vi "Begin.vi"(8 "error in":errorcluster) -> (0 "error out":errorcluster)   [LabVIEW 2014]
doc: "Called before other user functions, this VI is expected to open initial I/O refnums, load in file data, and do all program initialization. Notice that the <B>error out</B> terminal is simply used for data flow. Wiring it to other structures or subVIs ensures that this VI runs first."
uses:
  <vilib>/Rock Robotics/WPI/DriverStation/WPI_DriverStationRobotMode2.ctl
  <vilib>/Rock Robotics/WPI/Joystick/WPI_JoystickDeviceEnum.ctl
  <vilib>/Rock Robotics/WPI/Solenoid/WPI_SolenoidChannel.ctl
  <vilib>/Rock Robotics/SystemInterfaces/AI/FPGA_AIChannel.ctl
  <vilib>/Rock Robotics/SystemInterfaces/DIO/FPGA_DIOChannel.ctl
  <vilib>/Rock Robotics/WPI/CAN/TalonSRX/WPI_CANTalonSRX_APIControlMode.ctl
  <vilib>/Rock Robotics/WPI/CAN/TalonSRX/WPI_CANTalonSRX_BrakeOverride.ctl
  <vilib>/Rock Robotics/SystemInterfaces/i2clib/i2c_bus.ctl
  <vilib>/Rock Robotics/WPI/AnalogOutput/WPI_AnalogOutputChannel.ctl
  navX-MXP Library/COMMON/TypeDefs/Value TypeDefs/navX Update Rate.ctl
  navX-MXP Library/COMMON/TypeDefs/Value TypeDefs/navX Interface Protocol.ctl
  <vilib>/Rock Robotics/SystemInterfaces/spilib/spi_bus.ctl
  Robot Global Data.vi
  <vilib>/Rock Robotics/WPI/Solenoid/WPI_SolenoidOpenSingle.vi
  <vilib>/Rock Robotics/WPI/Counter/WPI_CounterDigitalInputToDigitalSource.vi
  <vilib>/Rock Robotics/WPI/MotorControl/WPI_MotorControlOpenCANTalonSRX.vi
  <vilib>/Rock Robotics/WPI/Ultrasonic/WPI_SonarSRF04DigitalOpen.vi
  <vilib>/Rock Robotics/WPI/Ultrasonic/WPI_SonarSRF04DigitalRefNum Registry Set.vi
  <vilib>/Rock Robotics/WPI/Compressor/WPI_CompressorGetSetRefNum.vi
  <vilib>/Rock Robotics/WPI/Camera/WPI_CameraWhite Balance Values.ctl
  <vilib>/Rock Robotics/WPI/Camera/WPI_CameraExposure Values.ctl
  <vilib>/Rock Robotics/WPI/Accelerometer/ADXL345 Range.ctl
  <vilib>/Rock Robotics/WPI/Accelerometer/WPI_AccelerometerADXL345 Axes.ctl
  <vilib>/Rock Robotics/WPI/RobotDrive/WPI_RobotDriveOpen2MotorWithExistingMotors.vi
  navX-MXP Library/navX-MXP IMU.lvlib
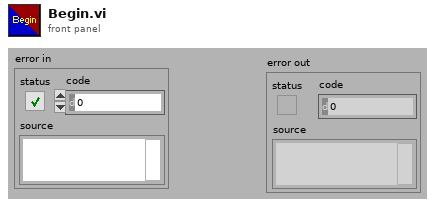
[diagram p1: front panel]
types:
  T1 = typedef "FPGA_DIOChannel.ctl" = enum8{"DIO 0", "DIO 1", "DIO 2", "DIO 3", "DIO 4", "DIO 5", "DIO 6", "DIO 7", "DIO 8", "DIO 9", "DIO MXP 0", "DIO MXP 1", "DIO MXP 2", "DIO MXP 3", "DIO MXP 4", "DIO MXP 5", "DIO MXP 6", "DIO MXP 7", "DIO MXP 8", "DIO MXP 9", "DIO MXP 10", "DIO MXP 11", "DIO MXP 12", "DIO MXP 13", "DIO MXP 14", "DIO MXP 15", "Invalid"}
  T2 = typedef "WPI_AnalogOutputChannel.ctl" = enum8{"AO MXP 0", "AO MXP 1", "Invalid"}
  T3 = typedef "i2c_bus.ctl" = enum16{"I2C On-Board", "I2C MXP", "Invalid"}
  T4 = typedef "FPGA_AIChannel.ctl" = enum8{"AI 0", "AI 1", "AI 2", "AI 3", "AI MXP 0", "AI MXP 1", "AI MXP 2", "AI MXP 3", "Invalid"}
  T5 = typedef "WPI_SolenoidChannel.ctl" = enum8{"Solenoid 0", "Solenoid 1", "Solenoid 2", "Solenoid 3", "Solenoid 4", "Solenoid 5", "Solenoid 6", "Solenoid 7", "Invalid"}
  T6 = typedef "WPI_CANTalonSRX_BrakeOverride.ctl" = enum8{"No Override", "Override to Coast", "Override to Brake"}
  T7 = typedef "WPI_CANTalonSRX_APIControlMode.ctl" = enum8{"Percent VBus", "Speed", "Position", "Slave", "Unchanged / Invalid"}
  T8 = typedef "WPI_JoystickDeviceEnum.ctl" = enum16{"USB 0", "USB 1", "USB 2", "USB 3", "USB 4", "USB 5"}
  T9 = typedef "WPI_DriverStationRobotMode2.ctl" = enum16{"Autonomous Disabled", "Autonomous Enabled", "Teleop Disabled", "Teleop Enabled", "Disconnected", "Finish", "Test Disabled", "Test Enabled", "Emergency Stopped"}
  T10 = typedef "WPI_CameraExposure Values.ctl" = enum16{"Auto", "Flicker-free 50 Hz", "Flicker-free 60 Hz", "Hold current", "Custom"}
  T11 = typedef "WPI_CameraWhite Balance Values.ctl" = enum16{"Auto", "Fixed indoor", "Fixed outdoor 1", "Fixed outdoor 2", "Fixed fluorescent 1", "Fixed fluorescent 2", "Hold current", "Custom"}
  T12 = typedef "WPI_CameraDevRef.ctl" = cluster{"Camera Address":string, "CameraStatus":errorcluster}
  T13 = typedef "WPI_SolenoidDevRef.ctl" = cluster{"DevStatus":errorcluster, "Pneumatics Control Module":u8, "Forward Solenoid Channel":T5, "Reverse Solenoid Channel":T5}
  T14 = typedef "WPI_MotorControlDeviceRef.ctl" = cluster{"DeviceStatus":errorcluster, "Type":T15, "PWM":cluster{"Controller":T16, "PWM Channel":T17, "DeadBand":T18}, "CAN":cluster{"Device Number":u8, "Control Mode":T19, "Semaphore":T20, "Max Vout":dbl, "TalonSRX Control Mode":T7}, "Invert":bool, "TransformRef":T21, "InvTransformRef":T21}
  T15 = typedef "WPI_MotorControlType.ctl" = enum16{"PWM", "CAN", "CANTalonSRX"}
  T16 = typedef "FPGA_TypedefDigitalModule.ctl" = enum16{"Controller 1"}
  T17 = typedef "FPGA_DIOPWMChannel.ctl" = enum8{"PWM 0", "PWM 1", "PWM 2", "PWM 3", "PWM 4", "PWM 5", "PWM 6", "PWM 7", "PWM 8", "PWM 9", "PWM MXP 0", "PWM MXP 1", "PWM MXP 2", "PWM MXP 3", "PWM MXP 4", "PWM MXP 5", "PWM MXP 6", "PWM MXP 7", "PWM MXP 8", "PWM MXP 9", "Invalid"}
  T18 = typedef "WPI_PWMDeadband.ctl" = cluster{"Name":string, "maxPositivePwm":i32, "minPositivePwm":i32, "centerPwm":i32, "maxNegativePwm":i32, "minNegativePwm":i32, "angularRange":u16}
  T19 = typedef "WPI_CANJaguar_ControlMode.ctl" = enum8{"Percent VBus", "Current", "Speed", "Position", "Voltage"}
  T20 = typedef "Semaphore RefNum" = refnum<k1>
  T21 = typedef "WPI_PWMTransform_ConPane.ctl" = refnum<vi>
  T22 = typedef "WPI_DigitalInputDevRef.ctl" = cluster{"DevStatus":errorcluster, "DIO Channel":T1, "Controller":T16}
  T23 = typedef "WPI_CompressorDevRef.ctl" = cluster{"DevStatus":errorcluster, "Pneumatics Control Module":u8}
  T24 = typedef "FPGA_CounterEncoderSourceConvertionLVSourceType.ctl" = cluster{"DevStatus":errorcluster, "AnalogTriggerMode?":bool, "DigitalMode":cluster{"Controller":T16, "DIO Channel":T25}, "AnalogTriggerMode":cluster{"AnalogTriggerIndex":T26, "OutputType":T27}}
  T25 = typedef "FPGA_DIODigitalSourceChannel.ctl" = enum8{"DIO 0", "DIO 1", "DIO 2", "DIO 3", "DIO 4", "DIO 5", "DIO 6", "DIO 7", "DIO 8", "DIO 9", "DIO MXP 0", "DIO MXP 1", "DIO MXP 2", "DIO MXP 3", "DIO MXP 4", "DIO MXP 5", "DIO MXP 6", "DIO MXP 7", "DIO MXP 8", "DIO MXP 9", "DIO MXP 10", "DIO MXP 11", "DIO MXP 12", "DIO MXP 13", "DIO MXP 14", "DIO MXP 15", "Disabled"}
  T26 = typedef "FPGA_AnalogTriggerIndex.ctl" = enum8{"Trig 0", "Trig 1", "Trig 2", "Trig 3", "Trig 4", "Trig 5", "Trig 6", "Trig 7", "Invalid"}
  T27 = typedef "FPGA_AnalogTriggerOutType.ctl" = enum16{"InWindow", "TriggerState", "Rising", "Falling"}
  T28 = typedef "WPI_EncoderDevRef.ctl" = cluster{"DevStatus":errorcluster, "EncoderIndex":T29, "CounterIndex":T30, "DistancePerCount":dbl, "Decoding Type":T31}
  T29 = typedef "FPGA_EncoderIdx.ctl" = enum8{"Enc 0", "Enc 1", "Enc 2", "Enc 3", "Enc 4", "Enc 5", "Enc 6", "Enc 7", "Invalid"}
  T30 = typedef "FPGA_CounterCtrSystemIndex.ctl" = enum8{"Ctr 0", "Ctr 1", "Ctr 2", "Ctr 3", "Ctr 4", "Ctr 5", "Ctr 6", "Ctr 7", "Invalid"}
  T31 = typedef "WPI_EncoderType.ctl" = enum16{"1x", "2x", "4x"}
  T32 = typedef "WPI_AccelerometerADXL345 Axes.ctl" = cluster{"X-Axis":bool, "Y-Axis":bool, "Z-Axis":bool}
  T33 = typedef "spi_bus.ctl" = enum16{"SPI On-Board, CS0", "SPI On-Board, CS1", "SPI On-Board, CS2", "SPI On-Board, CS3", "SPI MXP", "Invalid"}
  T34 = typedef "navX-MXP IMU.lvlib/navX Interface Protocol.ctl" = enum16{"SPI", "I2C"}
  T35 = typedef "navX-MXP IMU.lvlib/navX Update Rate.ctl" = u8
  T36 = typedef "WPI_I2CDevRef.ctl" = cluster{"DevStatus":errorcluster, "Controller":T16, "Device Address":u8, "Handle":i32, "I2C Bus":T3}
  T37 = typedef "ADXL345 Range.ctl" = u8
  T38 = typedef "WPI_AccelerometerDevRef.ctl" = cluster{"DevStatus":errorcluster, "Controller":T39, "Scaling":T40, "Analog Channels":T41, "I2C Bus":T3, "SPI Bus":T33, "Accel Range":T37, "ADXL345 Axes":T32, "Handle":i32, "Device Address":u8, "Accel Type":enum16{"Analog", "ADXL345 I2C", "ADXL345 SPI", "Internal"}}
  T39 = typedef "FPGA_TypedefAnalogModule.ctl" = enum16{"Controller 1"}
  T40 = typedef "WPI_AccelerometerScaling.ctl" = cluster{"Gain (VoltsPerG)":dbl, "Center Voltage":dbl}
  T41 = typedef "WPI_AccelerometerAnalogChannels.ctl" = cluster{"X-Axis":T4, "Y-Axis":T4, "Z-Axis":T4}
  T42 = typedef "navX-MXP IMU.lvlib/navX Device TypeDef.ctl" = cluster{"navX Interface Protocol":T34, "navX Interface Protocol TypeDefs":cluster{"SPIDevRef":T43, "I2CDevRef":T36}, "navX System Information":cluster{"Board Information":T44, "Status":T45, "Offsets":T49}, "navX Common Information":cluster{"Update Rate (4Hz-60Hz)":T35, "refnum name":string, "error":errorcluster}}
  T43 = typedef "WPI_SPIDevRef.ctl" = cluster{"DevStatus":errorcluster, "Handle":i32, "Controller":T16, "SPI Bus":T33}
  T44 = typedef "navX-MXP IMU.lvlib/navX Board Information.ctl" = cluster{"WhoAmI (50 | 0x32)":u8, "Board Revision":u8, "Firmware Major Version":u8, "Firmware Minor Version":u8}
  T45 = typedef "navX-MXP IMU.lvlib/navX Status Data.ctl" = cluster{"Update Rate Hz":u8, "Accelerometer Full-Scale Range":u8, "Gyro Full-Scale Range":u16, "NAVX_OP_STATUS":T46, "NAVX_CAL_STATUS":T47, "NAVX_SELFTEST_STATUS":u8, "NAVX_SENSOR_STATUS":T48}
  T46 = typedef "navX-MXP IMU.lvlib/navX NAVX_OP_STATUS.ctl" = u8
  T47 = typedef "navX-MXP IMU.lvlib/navX NAVX_CAL_STATUS.ctl" = u8
  T48 = typedef "navX-MXP IMU.lvlib/navX NAVX_SENSOR_STATUS.ctl" = cluster{"MOVING":bool, "YAW_STABLE":bool, "MAG_DISTURBANCE":bool, "ALTITUDE_VALID":bool, "SEALEVEL_PRESS_SET":bool, "FUSED_HEADING_VALID":bool}
  T49 = typedef "navX-MXP IMU.lvlib/navX Offsets Data.ctl" = cluster{"Yaw":dbl, "Quat W":dbl, "Quat X":dbl, "Quat Y":dbl, "Quat Z":dbl}
  T50 = typedef "WPI_AnalogChannelDevRef.ctl" = cluster{"DevStatus":errorcluster, "Controller":T39, "Analog Channel":T4}
  T51 = typedef "WPI_PotentiometerDevRef.ctl" = cluster{"DevStatus":errorcluster, "Controller":T39, "Analog Channel":T4, "Invert Output":bool}
  T52 = typedef "WPI_JoystickDevRef.ctl" = cluster{"Device":T8}
  T53 = typedef "WPI_RobotDriveDevRef.ctl" = cluster{"DevStatus":errorcluster, "Motors[]":T14[], "Square Inputs":bool, "Max Output":dbl}
  T54 = typedef "WPI_UltrasonicDeviceRef.ctl" = cluster{"DevStatus":errorcluster, "Ping Digital Controller":T16, "Echo Digital Controller":T16, "Ping Channel":T1, "Echo Channel":T1, "CntIndex":T30}
  T55 = typedef "WPI_AOChannelDevRef.ctl" = cluster{"DevStatus":errorcluster, "Controller":T39, "AO Channel":T2}
  T56 = typedef "WPI_DigitalOutputDevRef.ctl" = cluster{"Controller":T16, "DIO Channel":T1, "DevStatus":errorcluster}
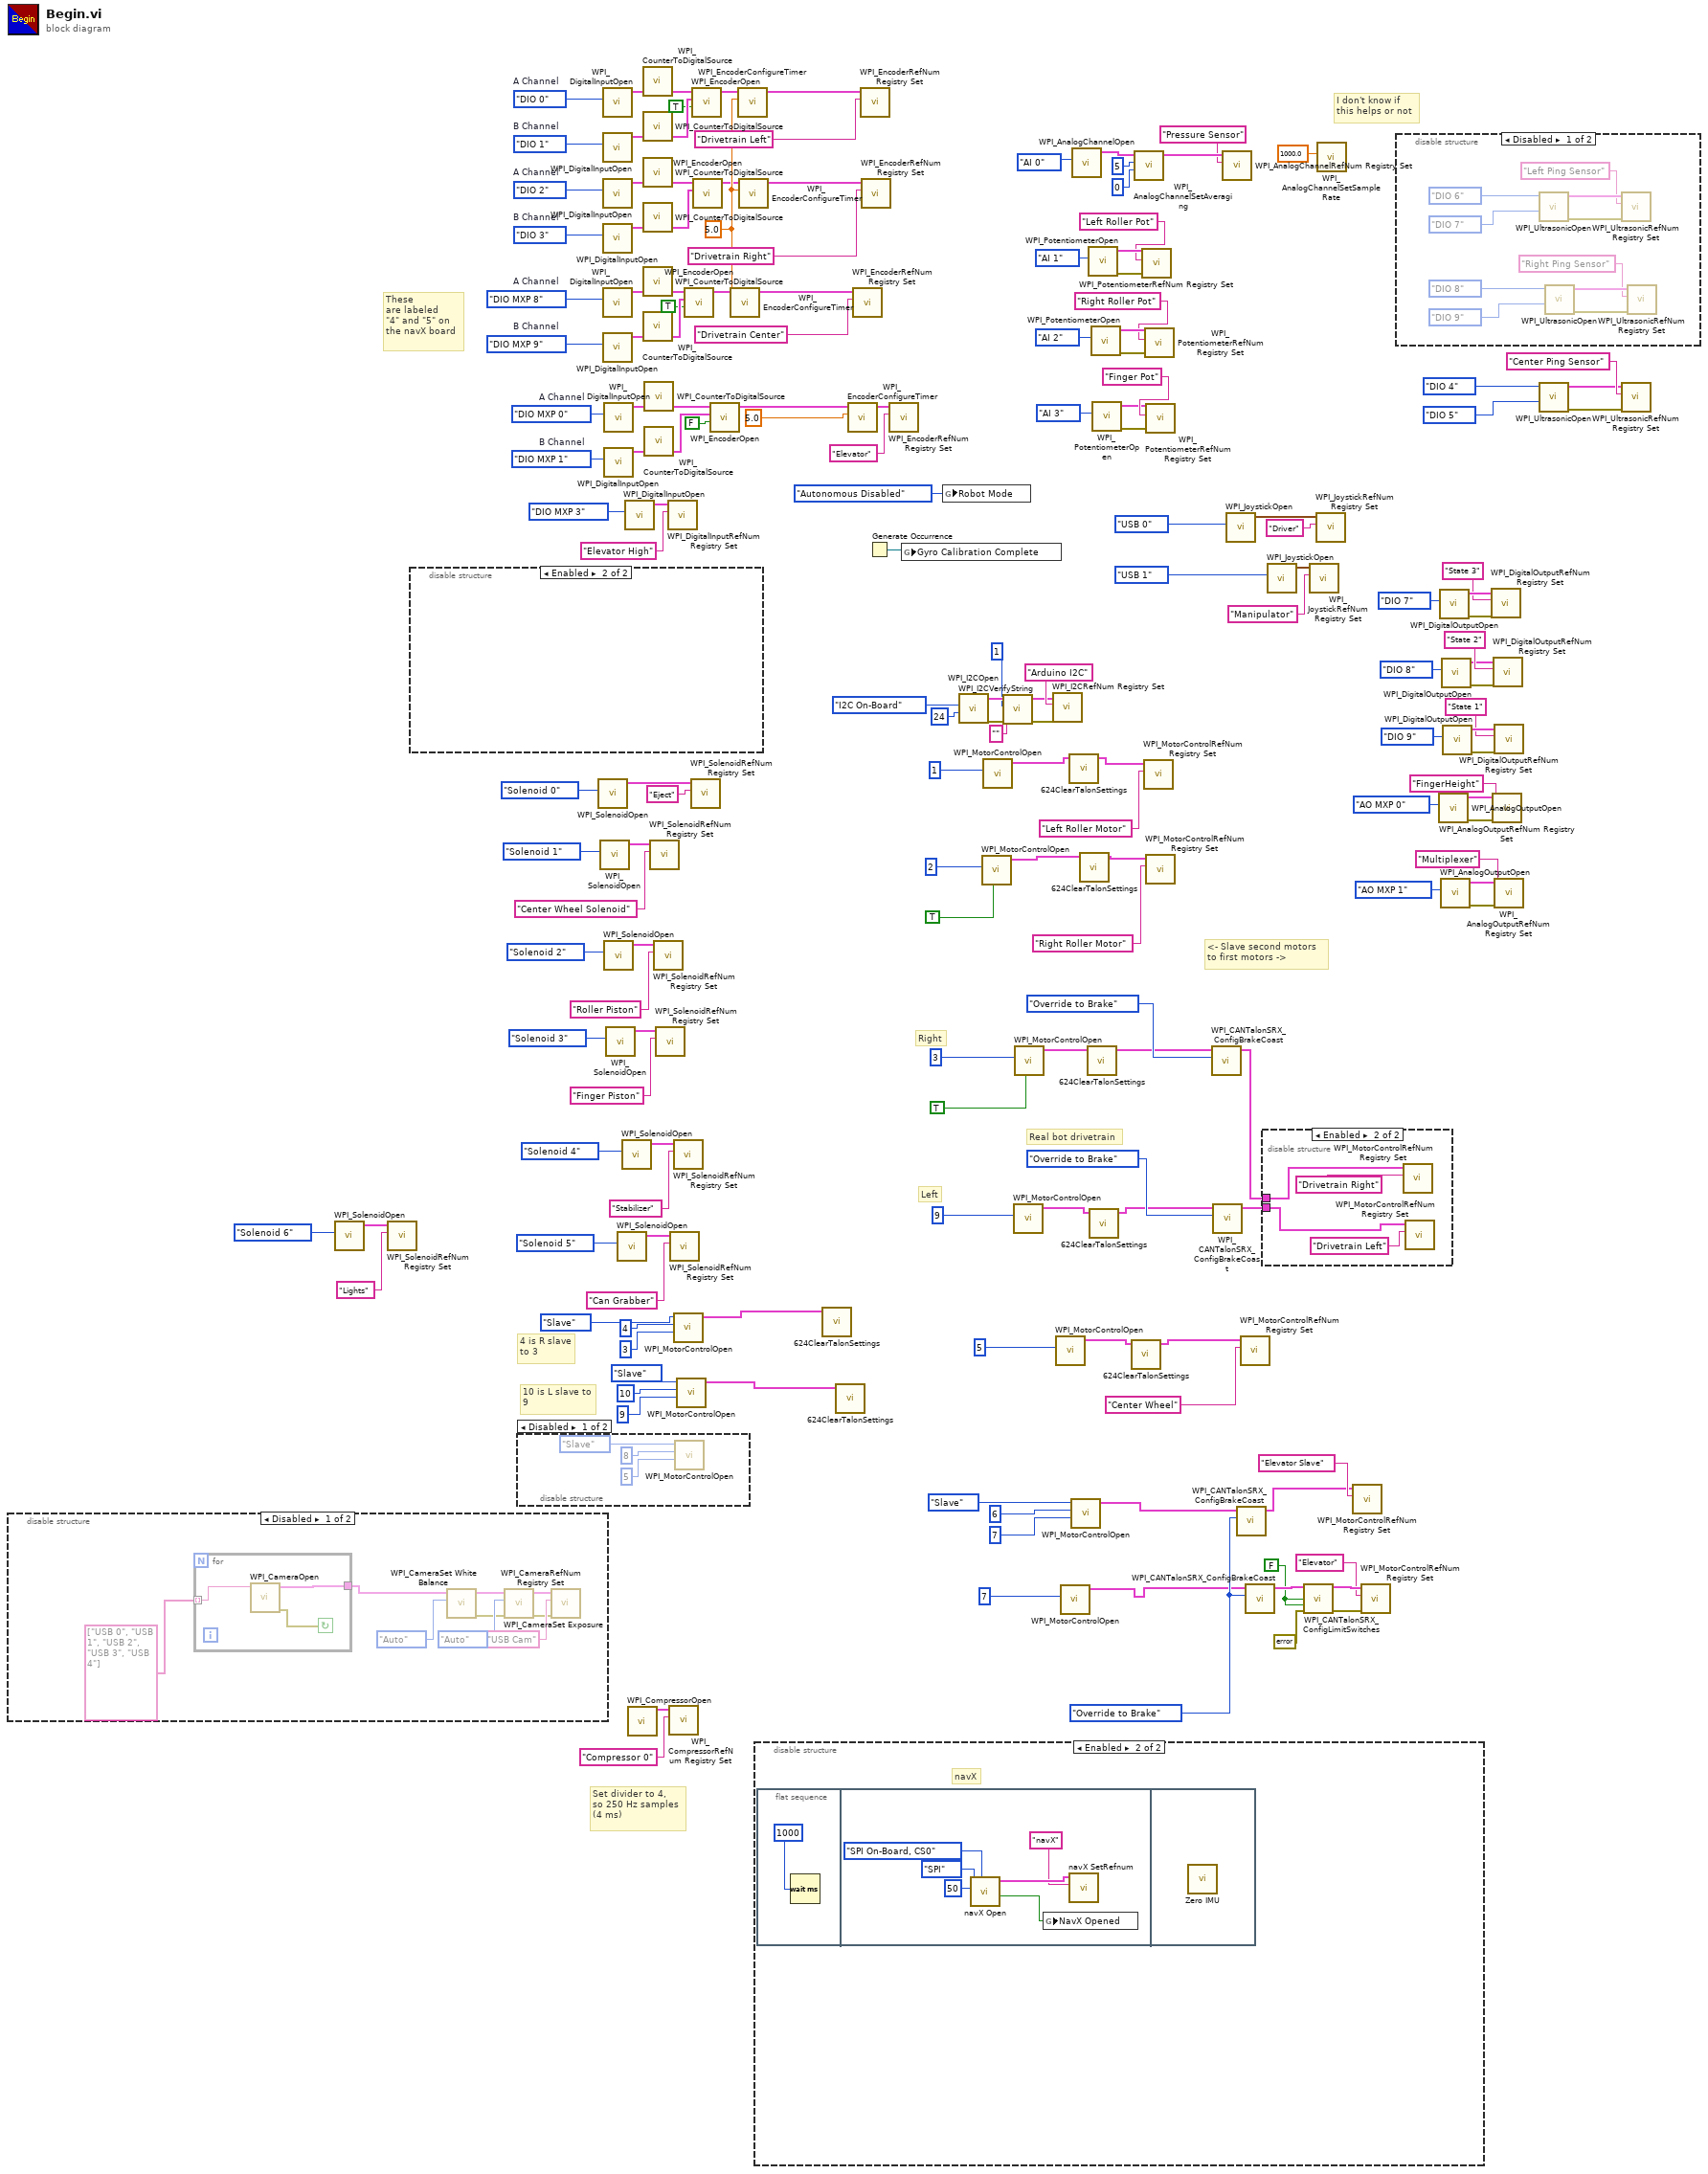
[diagram p0: block diagram]
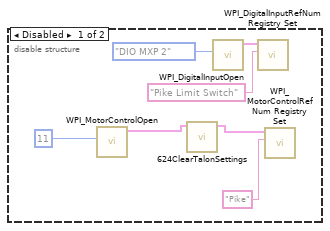
[diagram p2: hidden frame]
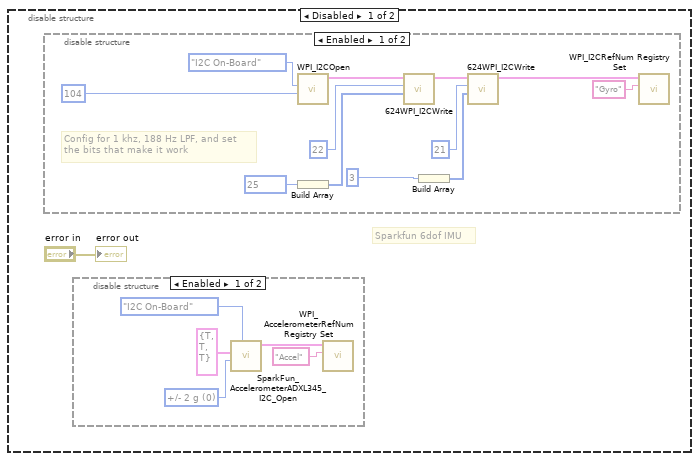
[diagram p5: hidden frame]
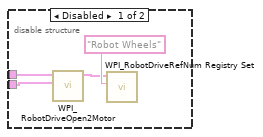
[diagram p9: hidden frame]
diagram:
  w37 = FPGA_DIOChannel."DIO MXP 9"  # B Channel
  w38 = FPGA_DIOChannel."DIO MXP 8"  # A Channel
  w62 = FALSE ("Forward Limit Switch Normally Open")
  w60 = WPI_CANTalonSRX_BrakeOverride."Override to Brake" ("Brake / Coast Mode")
  w90 = FPGA_DIOChannel."DIO MXP 1"  # B Channel
  w91 = FPGA_DIOChannel."DIO MXP 0"  # A Channel
  w118 = FPGA_DIOChannel."DIO 3"  # B Channel
  w121 = FPGA_DIOChannel."DIO 2"  # A Channel
  w127 = FPGA_DIOChannel."DIO 0"  # A Channel
  w130 = FPGA_DIOChannel."DIO 1"  # B Channel
  w135 = 5.0 ("Minimum Rate")
  # "10 is L slave to\n9"
  # "4 is R slave\nto 3"
  # "These \nare labeled\n\"4\" and \"5\" on \nthe navX board"
  # "<- Slave second motors\nto first motors ->"
  # "Left"
  # "Right"
  # "Real bot drivetrain"
  # "I don't know if \nthis helps or not"
  # "Set divider to 4, \nso 250 Hz samples\n(4 ms)"
  n1 = disable-structure shown="Disabled" {
    frame Disabled {
      n2 = for {
        tunnel: string[] ["USB 0", "USB 1", "USB 2", "USB 3", "USB 4"] -> [w187] mode=indexing
        tunnel: [w186] -> w176
        stop <- w185 continue-if-true
        n3 = call <vilib>:"WPI_CameraOpen.vi"("Camera Address"=w187) -> ("error out"=w185:errorcluster, "CameraDevRef"=w186:T12)  [unwired: 9 in]
      }
      n4 = call <vilib>:"WPI_CameraSet White Balance.vi"("White Balance"=WPI_CameraWhite_Balance_Values."Auto", "CameraDevRef"=w176) -> ("error out"=w179:errorcluster, "CameraDevRef Out"=w183:T12)  [unwired: 8 in]
      n5 = call <vilib>:"WPI_CameraSet Exposure.vi"("error in (no error)"=w179, "Exposure"=WPI_CameraExposure_Values."Auto", "CameraDevRef"=w183) -> ("error out"=w178:errorcluster, "CameraDevRef Out"=w181:T12)  [unwired: 7 in]
      n6 = call <vilib>:"WPI_CameraRefNum Registry Set.vi"("error in (no error)"=w178, "refnum name"="USB Cam", "CameraDevRef"=w181) -> ()  [unwired: 7 in, 2 out]
    }
    frame Enabled {
    }
  }
  n7 = call-poly <vilib>:"WPI_SolenoidOpen.vi"("Solenoid Channel"=WPI_SolenoidChannel."Solenoid 6") -> ("SolenoidDevRef"=w35:T13)  [unwired: 9 in, 1 out]
  n8 = call <vilib>:"WPI_SolenoidRefNum Registry Set.vi"("refnum name"="Lights", "SolenoidDevRef"=w35) -> ()  [unwired: 8 in, 2 out]
  n9 = disable-structure shown="Enabled" {
    frame Disabled {
      n10 = call-poly <vilib>:"WPI_MotorControlOpen.vi"("Device Number"=u8 11) -> ("MotorControlDeviceRef"=w190:T14)  [unwired: 9 in, 1 out]
      n11 = call "624ClearTalonSettings.vi"("CAN Talon SRX Ref Out"=w190) -> ("CAN Talon SRX Ref Out 2"=w189:T14)  [unwired: 10 in]
      n12 = call <vilib>:"WPI_DigitalInputOpen.vi"("DIO Channel"=FPGA_DIOChannel."DIO MXP 2") -> ("DigitalInputDevRef"=w192:T22)  [unwired: 9 in, 1 out]
      n13 = call <vilib>:"WPI_DigitalInputRefNum Registry Set.vi"("refnum name"="Pike Limit Switch", "DigitalInputDevRef"=w192) -> ()  [unwired: 8 in, 2 out]
      n14 = call <vilib>:"WPI_MotorControlRefNum Registry Set.vi"("refnum name"="Pike", "MotorControlDevRef"=w189) -> ()  [unwired: 8 in, 2 out]
    }
    frame Enabled {
    }
  }
  n15 = disable-structure shown="Disabled" {
    frame Disabled {
      n16 = call-poly <vilib>:"WPI_MotorControlOpen.vi"("Master Device Number"=u8 5, "Device Number"=u8 8, "Control Mode"=WPI_CANTalonSRX_APIControlMode."Slave") -> ()  [unwired: 7 in, 2 out]
    }
    frame Enabled {
    }
  }
  n17 = call-poly <vilib>:"WPI_SolenoidOpen.vi"("Solenoid Channel"=WPI_SolenoidChannel."Solenoid 0") -> ("SolenoidDevRef"=w104:T13)  [unwired: 9 in, 1 out]
  n18 = call-poly <vilib>:"WPI_SolenoidOpen.vi"("Solenoid Channel"=WPI_SolenoidChannel."Solenoid 1") -> ("SolenoidDevRef"=w103:T13)  [unwired: 9 in, 1 out]
  n19 = call <vilib>:"WPI_DigitalInputOpen.vi"("DIO Channel"=w127) -> ("DigitalInputDevRef"=w128:T22)  [unwired: 2 in, 8 out]
  n20 = call <vilib>:"WPI_DigitalInputOpen.vi"("DIO Channel"=w130) -> ("DigitalInputDevRef"=w131:T22)  [unwired: 2 in, 8 out]
  n21 = call <vilib>:"WPI_DigitalInputOpen.vi"("DIO Channel"=w121) -> ("DigitalInputDevRef"=w122:T22)  [unwired: 2 in, 8 out]
  n22 = call <vilib>:"WPI_DigitalInputOpen.vi"("DIO Channel"=w118) -> ("DigitalInputDevRef"=w119:T22)  [unwired: 2 in, 8 out]
  n23 = call <vilib>:"WPI_DigitalInputOpen.vi"("DIO Channel"=w38) -> ("DigitalInputDevRef"=w136:T22)  [unwired: 2 in, 8 out]
  n24 = call <vilib>:"WPI_DigitalInputOpen.vi"("DIO Channel"=w37) -> ("DigitalInputDevRef"=w138:T22)  [unwired: 2 in, 8 out]
  n25 = call <vilib>:"WPI_DigitalInputOpen.vi"("DIO Channel"=w91) -> ("DigitalInputDevRef"=w152:T22)  [unwired: 2 in, 8 out]
  n26 = call <vilib>:"WPI_DigitalInputOpen.vi"("DIO Channel"=w90) -> ("DigitalInputDevRef"=w154:T22)  [unwired: 2 in, 8 out]
  n27 = call-poly <vilib>:"WPI_SolenoidOpen.vi"("Solenoid Channel"=WPI_SolenoidChannel."Solenoid 2") -> ("SolenoidDevRef"=w105:T13)  [unwired: 9 in, 1 out]
  n28 = call-poly <vilib>:"WPI_SolenoidOpen.vi"("Solenoid Channel"=WPI_SolenoidChannel."Solenoid 3") -> ("SolenoidDevRef"=w107:T13)  [unwired: 9 in, 1 out]
  n29 = call-poly <vilib>:"WPI_SolenoidOpen.vi"("Solenoid Channel"=WPI_SolenoidChannel."Solenoid 5") -> ("SolenoidDevRef"=w41:T13)  [unwired: 9 in, 1 out]
  n30 = call-poly <vilib>:"WPI_SolenoidOpen.vi"("Solenoid Channel"=WPI_SolenoidChannel."Solenoid 4") -> ("SolenoidDevRef"=w110:T13)  [unwired: 9 in, 1 out]
  n31 = call <vilib>:"WPI_DigitalInputOpen.vi"("DIO Channel"=FPGA_DIOChannel."DIO MXP 3") -> ("DigitalInputDevRef"=w160:T22)  [unwired: 9 in, 1 out]
  n32 = call <vilib>:"WPI_CompressorOpen.vi"() -> ("CompressorDevRef"=w169:T23)  [unwired: 14 in, 1 out]
  n33 = call-poly <vilib>:"WPI_CounterToDigitalSource.vi"("DigitalInputDevRef"=w128) -> ("Digital Source"=w129:T24)  [unwired: 6 out]
  n34 = call-poly <vilib>:"WPI_CounterToDigitalSource.vi"("DigitalInputDevRef"=w131) -> ("Digital Source"=w132:T24)  [unwired: 6 out]
  n35 = call-poly <vilib>:"WPI_CounterToDigitalSource.vi"("DigitalInputDevRef"=w122) -> ("Digital Source"=w123:T24)  [unwired: 6 out]
  n36 = call-poly <vilib>:"WPI_CounterToDigitalSource.vi"("DigitalInputDevRef"=w119) -> ("Digital Source"=w120:T24)  [unwired: 6 out]
  n37 = call-poly <vilib>:"WPI_CounterToDigitalSource.vi"("DigitalInputDevRef"=w136) -> ("Digital Source"=w137:T24)  [unwired: 6 out]
  n38 = call-poly <vilib>:"WPI_CounterToDigitalSource.vi"("DigitalInputDevRef"=w138) -> ("Digital Source"=w139:T24)  [unwired: 6 out]
  n39 = call-poly <vilib>:"WPI_CounterToDigitalSource.vi"("DigitalInputDevRef"=w152) -> ("Digital Source"=w153:T24)  [unwired: 6 out]
  n40 = call-poly <vilib>:"WPI_CounterToDigitalSource.vi"("DigitalInputDevRef"=w154) -> ("Digital Source"=w155:T24)  [unwired: 6 out]
  n41 = call <vilib>:"WPI_SolenoidRefNum Registry Set.vi"("refnum name"="Center Wheel Solenoid", "SolenoidDevRef"=w103) -> ()  [unwired: 8 in, 2 out]
  n42 = call <vilib>:"WPI_SolenoidRefNum Registry Set.vi"("refnum name"="Roller Piston", "SolenoidDevRef"=w105) -> ()  [unwired: 8 in, 2 out]
  n43 = call <vilib>:"WPI_SolenoidRefNum Registry Set.vi"("refnum name"="Finger Piston", "SolenoidDevRef"=w107) -> ()  [unwired: 8 in, 2 out]
  n44 = call <vilib>:"WPI_DigitalInputRefNum Registry Set.vi"("refnum name"="Elevator High", "DigitalInputDevRef"=w160) -> ()  [unwired: 8 in, 2 out]
  n45 = call <vilib>:"WPI_CompressorRefNum Registry Set.vi"("refnum name"="Compressor 0", "CompressorDevRef"=w169) -> ()  [unwired: 8 in, 2 out]
  n46 = call <vilib>:"WPI_SolenoidRefNum Registry Set.vi"("refnum name"="Can Grabber", "SolenoidDevRef"=w41) -> ()  [unwired: 8 in, 2 out]
  n47 = call <vilib>:"WPI_SolenoidRefNum Registry Set.vi"("refnum name"="Stabilizer", "SolenoidDevRef"=w110) -> ()  [unwired: 8 in, 2 out]
  n48 = call-poly <vilib>:"WPI_MotorControlOpen.vi"("Master Device Number"=u8 3, "Device Number"=u8 4, "Control Mode"=WPI_CANTalonSRX_APIControlMode."Slave") -> ("MotorControlDeviceRef"=w49:T14)  [unwired: 7 in, 1 out]
  n49 = call-poly <vilib>:"WPI_MotorControlOpen.vi"("Master Device Number"=u8 9, "Device Number"=u8 10, "Control Mode"=WPI_CANTalonSRX_APIControlMode."Slave") -> ("MotorControlDeviceRef"=w48:T14)  [unwired: 7 in, 1 out]
  n50 = call <vilib>:"WPI_EncoderOpen.vi"("Invert Direction (False)"=TRUE, "BSource"=w139, "ASource"=w137) -> ("EncoderDevRef"=w140:T28)  [unwired: 5 in, 3 out]
  n51 = call <vilib>:"WPI_SolenoidRefNum Registry Set.vi"("refnum name"="Eject", "SolenoidDevRef"=w104) -> ()  [unwired: 8 in, 2 out]
  n52 = call <vilib>:"WPI_EncoderOpen.vi"("Invert Direction (False)"=TRUE, "BSource"=w132, "ASource"=w129) -> ("EncoderDevRef"=w133:T28)  [unwired: 5 in, 3 out]
  n53 = call <vilib>:"WPI_EncoderOpen.vi"("BSource"=w120, "ASource"=w123) -> ("EncoderDevRef"=w124:T28)  [unwired: 6 in, 3 out]
  n54 = call <vilib>:"WPI_EncoderOpen.vi"("Invert Direction (False)"=FALSE, "BSource"=w155, "ASource"=w153) -> ("EncoderDevRef"=w156:T28)  [unwired: 5 in, 3 out]
  n55 = call <vilib>:"WPI_EncoderConfigureTimer.vi"("Minimum Rate"=w135, "EncoderDevRef"=w140) -> ("EncoderDevRef"=w141:T28)  [unwired: 8 in, 1 out]
  n56 = call <vilib>:"WPI_EncoderConfigureTimer.vi"("Minimum Rate"=w135, "EncoderDevRef"=w133) -> ("EncoderDevRef"=w134:T28)  [unwired: 8 in, 1 out]
  n57 = call <vilib>:"WPI_EncoderConfigureTimer.vi"("Minimum Rate"=w135, "EncoderDevRef"=w124) -> ("EncoderDevRef"=w125:T28)  [unwired: 8 in, 1 out]
  n58 = disable-structure shown="Enabled" {
    frame Disabled {
      # "Sparkfun 6dof IMU"
      n59 = disable-structure shown="Enabled" {
        frame Enabled {
          # "Config for 1 khz, 188 Hz LPF, and set\nthe bits that make it work"
          n60 = call <vilib>:"WPI_I2COpen.vi"("Device Address"=104, "I2C Bus"=i2c_bus."I2C On-Board") -> ("I2CDevRef"=w214:T36)  [unwired: 8 in, 1 out]
          n61 = Build Array(u8 25) -> (w211:u8[])
          n62 = call "624WPI_I2CWrite.vi"("I2CDataToSend"=w211, "I2CRegister"=u8 22, "I2CDevRef"=w214) -> ("I2CDevRef"=w215:T36)  [unwired: 7 in, 1 out]
          n63 = Build Array(u8 3) -> (w208:u8[])
          n64 = call "624WPI_I2CWrite.vi"("I2CDataToSend"=w208, "I2CRegister"=u8 21, "I2CDevRef"=w215) -> ("I2CDevRef"=w204:T36)  [unwired: 7 in, 1 out]
          n65 = call <vilib>:"WPI_I2CRefNum Registry Set.vi"("refnum name"="Gyro", "I2CDevRef"=w204) -> ()  [unwired: 8 in, 2 out]
        }
        frame Disabled {
        }
      }
      n66 = disable-structure shown="Enabled" {
        frame Enabled {
          w202 = T37 0 items=["+/- 2 g", "+/- 4 g", "+/- 8 g", "+/- 16 g"] ("Accel Range")
          n67 = call "SparkFun_AccelerometerADXL345_I2C_Open.vi"("I2C Bus"=i2c_bus."I2C On-Board", "Accel Range"=w202, "ADXL345 Axes"=T32 {"X-Axis"=TRUE, "Y-Axis"=TRUE, "Z-Axis"=TRUE}) -> ("AccelerometerDevRef"=w203:T38)  [unwired: 7 in, 1 out]
          n68 = call <vilib>:"WPI_AccelerometerRefNum Registry Set.vi"("refnum name"="Accel", "AccelerometerDevRef"=w203) -> ()  [unwired: 8 in, 2 out]
        }
        frame Disabled {
        }
      }
      "error out" <- "error in"
    }
    frame Enabled {
      # "navX"
      n69 = flat-sequence {
        frame #0 {
          n70 = Wait (ms)(milliseconds to wait=u32 1000) -> ()  [unwired: 1 out]
        }
        frame #1 {
          n71 = call "navX Open.vi"("SPI Bus"=spi_bus."SPI On-Board, CS0", "Update Rate (4Hz-60Hz)"=T35 50, "navX Interface Protocol"=navX_Interface_Protocol."SPI") -> ("Opened?"=w220:bool, "navX Device TypeDef"=w222:T42)  [unwired: 6 in, 1 out]
          n72 = global write "Robot Global Data.vi" "NavX Opened"(w220) -> ()
          n73 = call "navX SetRefnum.vi"("refnum name"="navX", "navX Device TypeDef"=w222) -> ()  [unwired: 8 in, 2 out]
        }
        frame #2 {
          n74 = call "Zero IMU.vi"() -> ()  [unwired: 12 in]
        }
      }
    }
  }
  n75 = call "624ClearTalonSettings.vi"("CAN Talon SRX Ref Out"=w49) -> ()  [unwired: 10 in, 1 out]
  n76 = call "624ClearTalonSettings.vi"("CAN Talon SRX Ref Out"=w48) -> ()  [unwired: 10 in, 1 out]
  n77 = call <vilib>:"WPI_EncoderConfigureTimer.vi"("Minimum Rate"=5.0, "EncoderDevRef"=w156) -> ("EncoderDevRef"=w157:T28)  [unwired: 8 in, 1 out]
  n78 = call <vilib>:"WPI_EncoderRefNum Registry Set.vi"("refnum name"="Drivetrain Center", "EncoderDevRef"=w141) -> ()  [unwired: 8 in, 2 out]
  n79 = call <vilib>:"WPI_EncoderRefNum Registry Set.vi"("refnum name"="Drivetrain Left", "EncoderDevRef"=w134) -> ()  [unwired: 8 in, 2 out]
  n80 = call <vilib>:"WPI_EncoderRefNum Registry Set.vi"("refnum name"="Drivetrain Right", "EncoderDevRef"=w125) -> ()  [unwired: 8 in, 2 out]
  n81 = Generate Occurrence() -> (w44:refnum<k4>)
  n82 = call <vilib>:"WPI_EncoderRefNum Registry Set.vi"("refnum name"="Elevator", "EncoderDevRef"=w157) -> ()  [unwired: 8 in, 2 out]
  n83 = global write "Robot Global Data.vi" "Gyro Calibration Complete"(w44) -> ()
  n84 = global write "Robot Global Data.vi" "Robot Mode"(WPI_DriverStationRobotMode2."Autonomous Disabled" ("Robot Mode")) -> ()
  n85 = call <vilib>:"WPI_I2COpen.vi"("Device Address"=u8 24, "I2C Bus"=i2c_bus."I2C On-Board") -> ("error out"=w23:errorcluster, "I2CDevRef"=w26:T36)  [unwired: 8 in]
  n86 = call-poly <vilib>:"WPI_MotorControlOpen.vi"("Invert"=TRUE, "Device Number"=u8 2) -> ("MotorControlDeviceRef"=w52:T14)  [unwired: 8 in, 1 out]
  n87 = call-poly <vilib>:"WPI_MotorControlOpen.vi"("Device Number"=u8 1) -> ("MotorControlDeviceRef"=w50:T14)  [unwired: 9 in, 1 out]
  n88 = call <vilib>:"WPI_I2CVerifyString.vi"("error in (no error)"=w23, "Expected"="", "Register Address"=u8 1, "I2CDevRef"=w26) -> ("error out"=w24:errorcluster, "I2CDevRef"=w25:T36)  [unwired: 6 in]
  n89 = call-poly <vilib>:"WPI_MotorControlOpen.vi"("Device Number"=u8 9) -> ("MotorControlDeviceRef"=w56:T14)  [unwired: 9 in, 1 out]
  n90 = call-poly <vilib>:"WPI_MotorControlOpen.vi"("Invert"=TRUE, "Device Number"=u8 3) -> ("MotorControlDeviceRef"=w54:T14)  [unwired: 8 in, 1 out]
  n91 = call <vilib>:"WPI_I2CRefNum Registry Set.vi"("error in (no error)"=w24, "refnum name"="Arduino I2C", "I2CDevRef"=w25) -> ()  [unwired: 7 in, 2 out]
  n92 = call-poly <vilib>:"WPI_MotorControlOpen.vi"("Device Number"=u8 5) -> ("MotorControlDeviceRef"=w58:T14)  [unwired: 9 in, 1 out]
  n93 = call-poly <vilib>:"WPI_MotorControlOpen.vi"("Device Number"=u8 7) -> ("MotorControlDeviceRef"=w45:T14)  [unwired: 9 in, 1 out]
  n94 = call "624ClearTalonSettings.vi"("CAN Talon SRX Ref Out"=w50) -> ("CAN Talon SRX Ref Out 2"=w51:T14)  [unwired: 10 in]
  n95 = call-poly <vilib>:"WPI_MotorControlOpen.vi"("Master Device Number"=u8 7, "Device Number"=u8 6, "Control Mode"=WPI_CANTalonSRX_APIControlMode."Slave") -> ("MotorControlDeviceRef"=w46:T14)  [unwired: 7 in, 1 out]
  n96 = call <vilib>:"WPI_AnalogChannelOpen.vi"("Analog Channel"=FPGA_AIChannel."AI 0") -> ("AIDeviceRef"=w165:T50)  [unwired: 9 in, 1 out]
  n97 = call "624ClearTalonSettings.vi"("CAN Talon SRX Ref Out"=w52) -> ("CAN Talon SRX Ref Out 2"=w53:T14)  [unwired: 10 in]
  n98 = call "624ClearTalonSettings.vi"("CAN Talon SRX Ref Out"=w54) -> ("CAN Talon SRX Ref Out 2"=w55:T14)  [unwired: 10 in]
  n99 = call <vilib>:"WPI_PotentiometerOpen.vi"("Analog Channel"=FPGA_AIChannel."AI 1") -> ("error out"=w95:errorcluster, "PotDevRef"=w94:T51)  [unwired: 9 in]
  n100 = call "624ClearTalonSettings.vi"("CAN Talon SRX Ref Out"=w56) -> ("CAN Talon SRX Ref Out 2"=w57:T14)  [unwired: 10 in]
  n101 = call <vilib>:"WPI_PotentiometerOpen.vi"("Analog Channel"=FPGA_AIChannel."AI 2") -> ("error out"=w99:errorcluster, "PotDevRef"=w98:T51)  [unwired: 9 in]
  n102 = call <vilib>:"WPI_PotentiometerOpen.vi"("Analog Channel"=FPGA_AIChannel."AI 3") -> ("error out"=w30:errorcluster, "PotDevRef"=w31:T51)  [unwired: 9 in]
  n103 = call "624ClearTalonSettings.vi"("CAN Talon SRX Ref Out"=w58) -> ("CAN Talon SRX Ref Out 2"=w59:T14)  [unwired: 10 in]
  n104 = call <vilib>:"WPI_AnalogChannelSetAveraging.vi"("OversampleBits"=u8 0, "AverageBits"=u8 5, "AIDeviceRef"=w165) -> ("AIDeviceRef"=w166:T50)  [unwired: 7 in, 1 out]
  n105 = call <vilib>:"WPI_PotentiometerRefNum Registry Set.vi"("error in (no error)"=w95, "refnum name"="Left Roller Pot", "PotDevRef"=w94) -> ()  [unwired: 7 in, 2 out]
  n106 = call <vilib>:"WPI_MotorControlRefNum Registry Set.vi"("refnum name"="Left Roller Motor", "MotorControlDevRef"=w51) -> ()  [unwired: 8 in, 2 out]
  n107 = call <vilib>:"WPI_PotentiometerRefNum Registry Set.vi"("error in (no error)"=w99, "refnum name"="Right Roller Pot", "PotDevRef"=w98) -> ()  [unwired: 7 in, 2 out]
  n108 = call <vilib>:"WPI_PotentiometerRefNum Registry Set.vi"("error in (no error)"=w30, "refnum name"="Finger Pot", "PotDevRef"=w31) -> ()  [unwired: 7 in, 2 out]
  n109 = call <vilib>:"WPI_MotorControlRefNum Registry Set.vi"("refnum name"="Right Roller Motor", "MotorControlDevRef"=w53) -> ()  [unwired: 8 in, 2 out]
  n110 = call <vilib>:"WPI_CANTalonSRX_ConfigBrakeCoast.vi"("Brake / Coast Mode"=WPI_CANTalonSRX_BrakeOverride."Override to Brake", "CAN Talon SRX Ref"=w55) -> ("CAN Talon SRX Ref Out"=w78:T14)  [unwired: 8 in, 1 out]
  n111 = call <vilib>:"WPI_CANTalonSRX_ConfigBrakeCoast.vi"("Brake / Coast Mode"=WPI_CANTalonSRX_BrakeOverride."Override to Brake", "CAN Talon SRX Ref"=w57) -> ("CAN Talon SRX Ref Out"=w81:T14)  [unwired: 8 in, 1 out]
  n112 = call <vilib>:"WPI_AnalogChannelRefNum Registry Set.vi"("refnum name"="Pressure Sensor", "AIDeviceRef"=w166) -> ()  [unwired: 8 in, 2 out]
  n113 = call <vilib>:"WPI_JoystickOpen.vi"("JoystickDevice"=WPI_JoystickDeviceEnum."USB 0") -> ("JoystickDevRef"=w174:T52)  [unwired: 10 in]
  n114 = call <vilib>:"WPI_CANTalonSRX_ConfigBrakeCoast.vi"("Brake / Coast Mode"=w60, "CAN Talon SRX Ref"=w46) -> ("CAN Talon SRX Ref Out"=w42:T14)  [unwired: 8 in, 1 out]
  n115 = call <vilib>:"WPI_MotorControlRefNum Registry Set.vi"("refnum name"="Center Wheel", "MotorControlDevRef"=w59) -> ()  [unwired: 8 in, 2 out]
  n116 = call <vilib>:"WPI_CANTalonSRX_ConfigBrakeCoast.vi"("Brake / Coast Mode"=w60, "CAN Talon SRX Ref"=w45) -> ("CAN Talon SRX Ref Out"=w64:T14)  [unwired: 8 in, 1 out]
  n117 = disable-structure shown="Enabled" {
    disable-tunnel: w81 -> [w224 w227]
    disable-tunnel: w78 -> [w223 w230]
    frame Disabled {
      n118 = call-poly <vilib>:"WPI_RobotDriveOpen2Motor.vi"("Right Motor Dev Ref"=w224, "Left Motor Dev Ref"=w223) -> ("RobotDriveDevRef"=w225:T53)  [unwired: 8 in, 1 out]
      n119 = call <vilib>:"WPI_RobotDriveRefNum Registry Set.vi"("refnum name"="Robot Wheels", "RobotDriveDevRef"=w225) -> ()  [unwired: 8 in, 2 out]
    }
    frame Enabled {
      n120 = call <vilib>:"WPI_MotorControlRefNum Registry Set.vi"("refnum name"="Drivetrain Right", "MotorControlDevRef"=w230) -> ()  [unwired: 8 in, 2 out]
      n121 = call <vilib>:"WPI_MotorControlRefNum Registry Set.vi"("refnum name"="Drivetrain Left", "MotorControlDevRef"=w227) -> ()  [unwired: 8 in, 2 out]
    }
  }
  n122 = call <vilib>:"WPI_JoystickOpen.vi"("JoystickDevice"=WPI_JoystickDeviceEnum."USB 1") -> ("JoystickDevRef"=w147:T52)  [unwired: 10 in]
  n123 = call <vilib>:"WPI_CANTalonSRX_ConfigLimitSwitches.vi"("CAN Talon SRX Ref"=w64, "Forward Limit Switch Normally Open"=w62, "Reverse Limit Switch Normally Open"=w62, "error in (no error)"=errorcluster {"status"=FALSE, "code"=0, "source"=""}) -> ("CAN Talon SRX Ref Out"=w66:T14, "error out"=w65:errorcluster)  [unwired: 10 in]
  n124 = call <vilib>:"WPI_JoystickRefNum Registry Set.vi"("refnum name"="Manipulator", "JoystickDevRef"=w147) -> ()  [unwired: 8 in, 2 out]
  n125 = call <vilib>:"WPI_JoystickRefNum Registry Set.vi"("refnum name"="Driver", "JoystickDevRef"=w174) -> ()  [unwired: 8 in, 2 out]
  n126 = call <vilib>:"WPI_AnalogChannelSetSampleRate.vi"("Samples Per Second (per channel)"=1000.0) -> ()  [unwired: 9 in, 2 out]
  n127 = call <vilib>:"WPI_MotorControlRefNum Registry Set.vi"("refnum name"="Elevator Slave", "MotorControlDevRef"=w42) -> ()  [unwired: 8 in, 2 out]
  n128 = call <vilib>:"WPI_MotorControlRefNum Registry Set.vi"("error in (no error)"=w65, "refnum name"="Elevator", "MotorControlDevRef"=w66) -> ()  [unwired: 7 in, 2 out]
  n129 = disable-structure shown="Disabled" {
    frame Disabled {
      n130 = call-poly <vilib>:"WPI_UltrasonicOpen.vi"("Echo DIO Channel"=FPGA_DIOChannel."DIO 7", "Ping DIO Channel"=FPGA_DIOChannel."DIO 6") -> ("error out"=w235:errorcluster, "SonarSRF04DevRef"=w234:T54)  [unwired: 8 in]
      n131 = call-poly <vilib>:"WPI_UltrasonicOpen.vi"("Echo DIO Channel"=FPGA_DIOChannel."DIO 9", "Ping DIO Channel"=FPGA_DIOChannel."DIO 8") -> ("error out"=w240:errorcluster, "SonarSRF04DevRef"=w239:T54)  [unwired: 8 in]
      n132 = call-poly <vilib>:"WPI_UltrasonicRefNum Registry Set.vi"("error in (no error)"=w235, "refnum name"="Left Ping Sensor", "SonarSRF04DevRef"=w234) -> ()  [unwired: 7 in, 2 out]
      n133 = call-poly <vilib>:"WPI_UltrasonicRefNum Registry Set.vi"("error in (no error)"=w240, "refnum name"="Right Ping Sensor", "SonarSRF04DevRef"=w239) -> ()  [unwired: 7 in, 2 out]
    }
    frame Enabled {
    }
  }
  n134 = call <vilib>:"WPI_AnalogOutputOpen.vi"("AO Channel"=WPI_AnalogOutputChannel."AO MXP 0") -> ("error out"=w15:errorcluster, "AODeviceRef"=w16:T55)  [unwired: 9 in]
  n135 = call <vilib>:"WPI_DigitalOutputOpen.vi"("DIO Channel"=FPGA_DIOChannel."DIO 7") -> ("error out"=w4:errorcluster, "DigitalOutputDevRef"=w3:T56)  [unwired: 9 in]
  n136 = call <vilib>:"WPI_AnalogOutputOpen.vi"("AO Channel"=WPI_AnalogOutputChannel."AO MXP 1") -> ("error out"=w13:errorcluster, "AODeviceRef"=w10:T55)  [unwired: 9 in]
  n137 = call <vilib>:"WPI_DigitalOutputOpen.vi"("DIO Channel"=FPGA_DIOChannel."DIO 8") -> ("error out"=w5:errorcluster, "DigitalOutputDevRef"=w6:T56)  [unwired: 9 in]
  n138 = call <vilib>:"WPI_DigitalOutputOpen.vi"("DIO Channel"=FPGA_DIOChannel."DIO 9") -> ("error out"=w20:errorcluster, "DigitalOutputDevRef"=w19:T56)  [unwired: 9 in]
  n139 = call <vilib>:"WPI_DigitalOutputRefNum Registry Set.vi"("error in (no error)"=w4, "refnum name"="State 3", "DigitalOutputDevRef"=w3) -> ()  [unwired: 7 in, 2 out]
  n140 = call <vilib>:"WPI_AnalogOutputRefNum Registry Set.vi"("error in (no error)"=w15, "refnum name"="FingerHeight", "AODeviceRef"=w16) -> ()  [unwired: 7 in, 2 out]
  n141 = call <vilib>:"WPI_DigitalOutputRefNum Registry Set.vi"("error in (no error)"=w5, "refnum name"="State 2", "DigitalOutputDevRef"=w6) -> ()  [unwired: 7 in, 2 out]
  n142 = call <vilib>:"WPI_DigitalOutputRefNum Registry Set.vi"("error in (no error)"=w20, "refnum name"="State 1", "DigitalOutputDevRef"=w19) -> ()  [unwired: 7 in, 2 out]
  n143 = call <vilib>:"WPI_AnalogOutputRefNum Registry Set.vi"("error in (no error)"=w13, "refnum name"="Multiplexer", "AODeviceRef"=w10) -> ()  [unwired: 7 in, 2 out]
  n144 = call-poly <vilib>:"WPI_UltrasonicOpen.vi"("Echo DIO Channel"=FPGA_DIOChannel."DIO 5", "Ping DIO Channel"=FPGA_DIOChannel."DIO 4") -> ("error out"=w70:errorcluster, "SonarSRF04DevRef"=w71:T54)  [unwired: 8 in]
  n145 = call-poly <vilib>:"WPI_UltrasonicRefNum Registry Set.vi"("error in (no error)"=w70, "refnum name"="Center Ping Sensor", "SonarSRF04DevRef"=w71) -> ()  [unwired: 7 in, 2 out]
